vi "DecodeSegmentSpecLine.vi"(8 "error in (no error)":errorcluster, 11 "Segment Spec Line":string) -> (0 "error out":errorcluster, 3 "Segment Spec Info":T1)   [LabVIEW 2012]
uses:
  #TD_SegmentSpecInfo.ctl
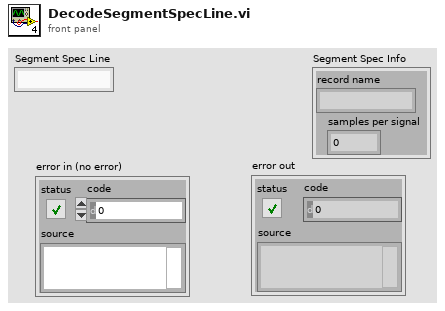
[diagram p1: front panel]
types:
  T1 = typedef "#TD_SegmentSpecInfo.ctl" = cluster{"record name":string, "samples per signal":i32}
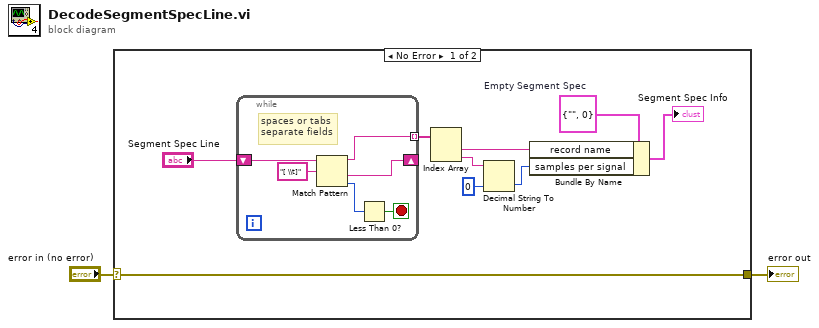
[diagram p0: block diagram]
diagram:
  n1 = case shown="No Error" "error in (no error)" {
    selector: "error in (no error)" -> [w3 w18]
    tunnel: [w3 w18] -> w1
    frame No Error {
      w7 = T1 {"record name"="", "samples per signal"=0}  # Empty Segment Spec
      n2 = while {
        shift-right: [w13] -> _
        shift-left: "Segment Spec Line" -> [w17]
        tunnel: [w12] -> w5 mode=indexing
        stop <- w15 stop-if-true
        # "spaces or tabs\nseparate fields"
        n3 = Match Pattern(string=w17, regular expression="[ \\t]") -> (before substring=w12:string, after substring=w13:string, offset past match=w16:i32)  [unwired: 1 in, 1 out]
        n4 = Less Than 0?(x=w16) -> (x < 0?=w15:bool)
      }
      n5 = Index Array(array=w5) -> (element #1=w10:string, element #2=w6:string)  [unwired: 2 in]
      n6 = Decimal String To Number(string=w6, default (0L)=0 ("default (0 I32)")) -> (number=w8:i32)  [unwired: 1 in, 1 out]
      n7 = Bundle By Name(cluster=w7, "record name"=w10, "samples per signal"=w8) -> (→"Segment Spec Info":T1)
    }
    frame Error {
    }
  }
  "error out" <- w1
